vi "Read target.vi"(8 "error in (no error)":errorcluster, 11 "SecMirror in":refnum<class "SecMirror.lvclass">) -> (0 "error out":errorcluster, 2 "target":i32, 3 "SecMirror out":refnum<class "SecMirror.lvclass">)   [LabVIEW 2018, in "SecMirror.lvclass"]
uses:
  SecMirror.lvclass
  SecMirror.lvclass/SecMirror.ctl
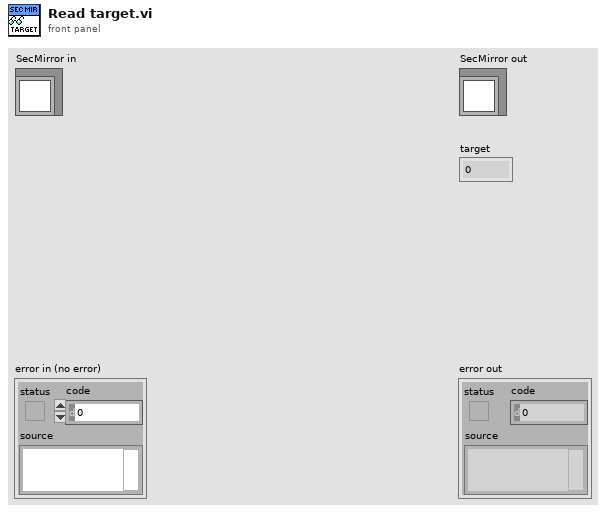
[diagram p1: front panel]
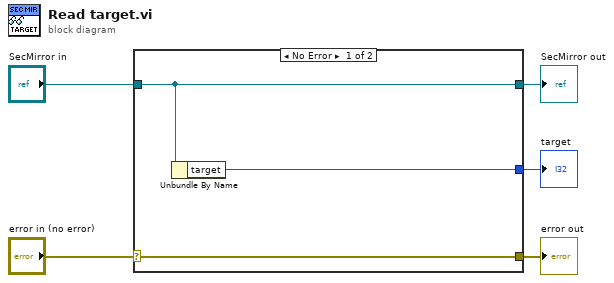
[diagram p0: block diagram]
diagram:
  n1 = case shown="No Error" "error in (no error)" {
    selector: "error in (no error)" -> [w8 w9]
    tunnel: [w8 w9] -> w4
    tunnel: [w7 w10] -> w2
    tunnel: "SecMirror in" -> [w7 w10]
    tunnel: [w6 _] -> w1
    frame No Error {
      n2 = Unbundle By Name(w7) -> ("target"=w6:i32)
    }
    frame Error {
    }
  }
  "error out" <- w4
  "SecMirror out" <- w2
  "target" <- w1
